vi "UpdateAnnulusROI.vi"(0 "Fitted Circle":T3, 1 "Circle fit parameters in":T2) -> (2 "Annulus Roi":T1, 3 "Pupil Found":bool, 4 "Circle fit parameters out":T2)   [LabVIEW 2013]
doc: "Updates Circle Fit parameters with the latest results from the circle fitting. Also outputs the coordinates for the fitted circle in the original image."
uses:
  TrackingParameters.ctl
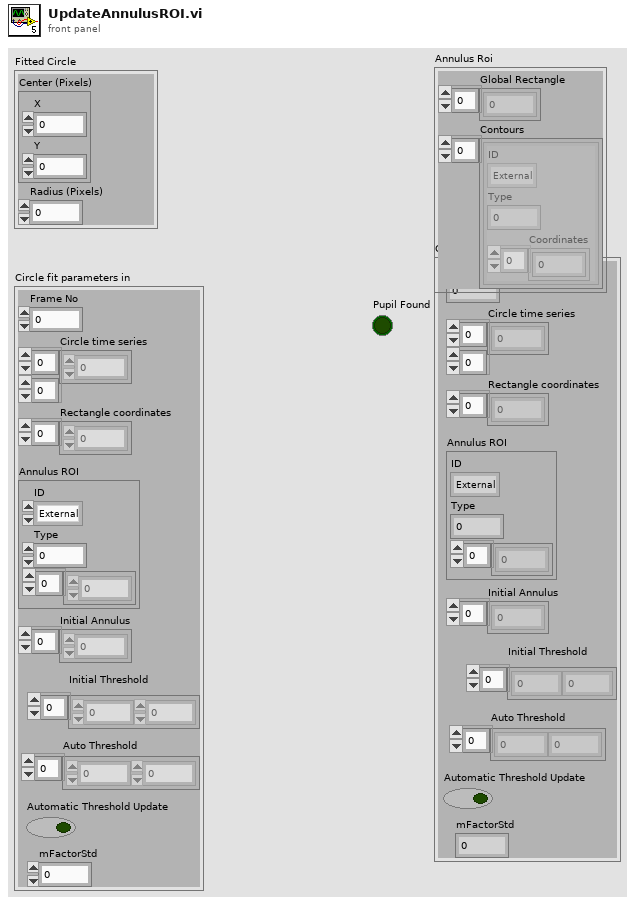
[diagram p1: front panel]
types:
  T1 = cluster{"Global Rectangle":i32[], "Contours":cluster{"ID":enum32{"External", "Internal"}, "Type":u32, "Coordinates":i32[]}[]}
  T2 = typedef "TrackingParameters.ctl" = cluster{"Frame No":i32, "Circle time series":dbl[][], "Rectangle coordinates":i32[], "Annulus ROI":cluster{"ID":enum32{"External", "Internal"}, "Type":u32, i32[]}, "Initial Annulus":i32[], "Auto Threshold":sgl[], "Automatic Threshold Update":bool, "Initial Threshold":sgl[], "mFactorStd":dbl}
  T3 = cluster{"Center (Pixels)":cluster{"X":sgl, "Y":sgl}, "Radius (Pixels)":dbl, "Center (Real-World)":cluster{"X":sgl, "Y":sgl}, "Radius (Real-World)":dbl, "Roundness (Real-World)":dbl, "Average Strength":dbl, "Average SNR (dB)":dbl}
  T4 = cluster{"ID":enum32{"External", "Internal"}, "Type":u32, i32[]}
  T5 = cluster{"ID":enum32{"External", "Internal"}, "Type":u32, i32[]}[]
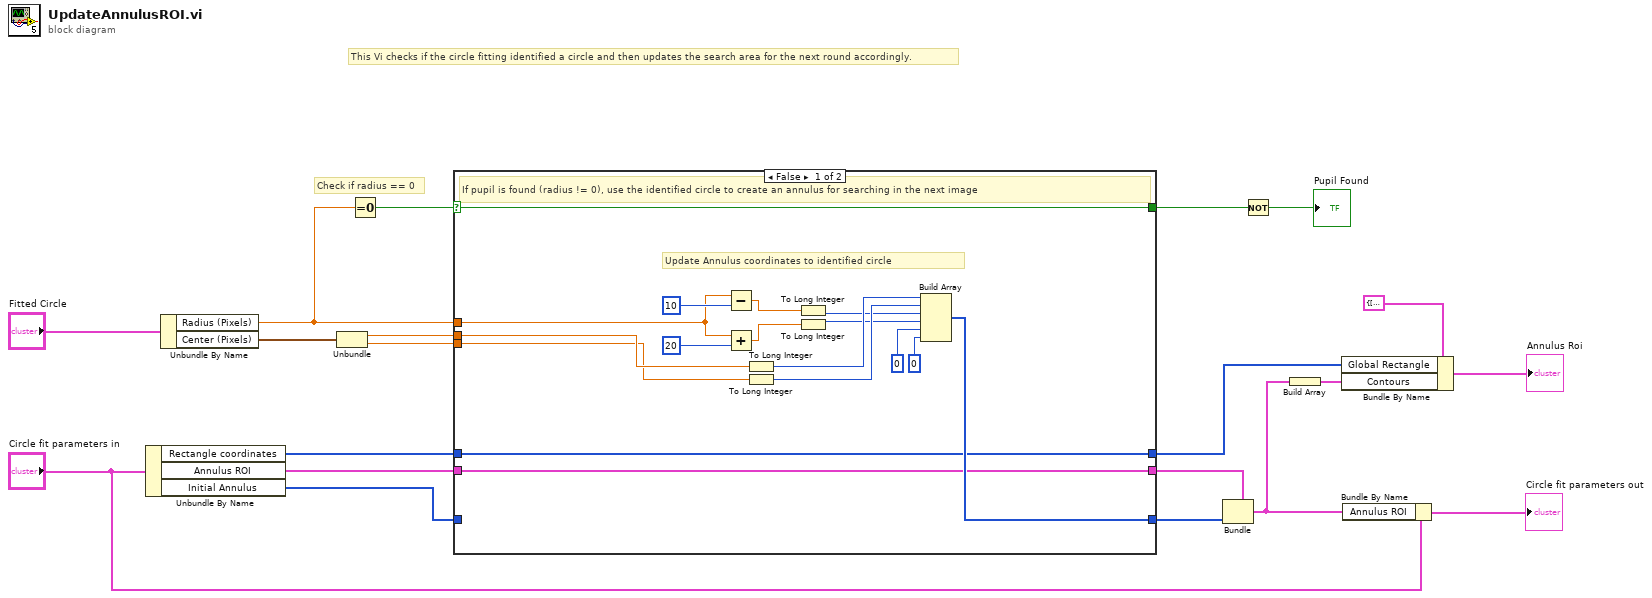
[diagram p0: block diagram]
diagram:
  # "This Vi checks if the circle fitting identified a circle and then updates the search area for the next round accordingly."
  # "Check if radius == 0"
  n1 = Unbundle By Name("Circle fit parameters in") -> ("Rectangle coordinates"=w3:i32[], "Annulus ROI"=w10:T4, "Initial Annulus"=w11:i32[])
  n2 = Unbundle By Name("Fitted Circle") -> ("Radius (Pixels)"=w9:dbl, "Center (Pixels)"=w19:cluster{"X":sgl, "Y":sgl})
  n3 = Unbundle(w19) -> ("X"=w17:sgl, "Y"=w16:sgl)
  n4 = Equal To 0?(x=w9) -> (x = 0?=w20:bool)
  n5 = case shown="False" w20 {
    selector: w20 -> [w22 w39]
    tunnel: w11 -> [_ w41]
    tunnel: [w31 w41] -> w13
    tunnel: w9 -> [w26 _]
    tunnel: w17 -> [w25 _]
    tunnel: w16 -> [w24 _]
    tunnel: w10 -> [w23 w40]
    tunnel: [w23 w40] -> w14
    tunnel: [w22 w39] -> w8
    tunnel: [w21 w38] -> w4
    tunnel: w3 -> [w21 w38]
    frame False {
      # "Update Annulus coordinates to identified circle"
      # "If pupil is found (radius != 0), use the identified circle to create an annulus for searching in the next image"
      n6 = Subtract(x=w26, y=10) -> (x-y=w30:dbl)
      n7 = Add(x=w26, y=20) -> (x+y=w28:dbl)
      n8 = To Long Integer(number=w25) -> (32bit integer=w37:i32)
      n9 = To Long Integer(number=w24) -> (32bit integer=w36:i32)
      n10 = To Long Integer(number=w30) -> (32bit integer=w29:i32)
      n11 = To Long Integer(number=w28) -> (32bit integer=w27:i32)
      n12 = Build Array(w37, w36, w29, w27, 0, 0) -> (w31:i32[])
    }
    frame True {
      # "If pupil is not found (radius=0), reset the annulus to initial, and use that for searching"
    }
  }
  n13 = Bundle(cluster=w14, w13) -> (w2:T4)  [unwired: 2 in]
  n14 = Not(x=w8) -> (.not. x?=→"Pupil Found":bool)
  n15 = Build Array(w2) -> (w1:T5)
  n16 = Bundle By Name(cluster=T1 {"Global Rectangle"=[63, 39, 363, 338], "Contours"=[{"ID"=enum."External", "Type"=7, "Coordinates"=[212, 188, 9, 149, 0, 0]}]} ("ROI Descriptor (Find Circular Edge 1)"), "Global Rectangle"=w4, "Contours"=w1) -> (→"Annulus Roi":T1)
  n17 = Bundle By Name(cluster="Circle fit parameters in", "Annulus ROI"=w2) -> (→"Circle fit parameters out":T2)
